vi "OEE_SCREEN_2_update_graph_accumulative_data.vi"(11 "SQL_raw_data_out":T1) -> ()   [LabVIEW 2019]
uses:
  FGV/SQL_raw_data/OEE_SQL_raw_data.ctl
  FGV/FGV_SCREEN_2_graph_accumulative/FGV_SCREEN_2_graph_accumulative.ctl
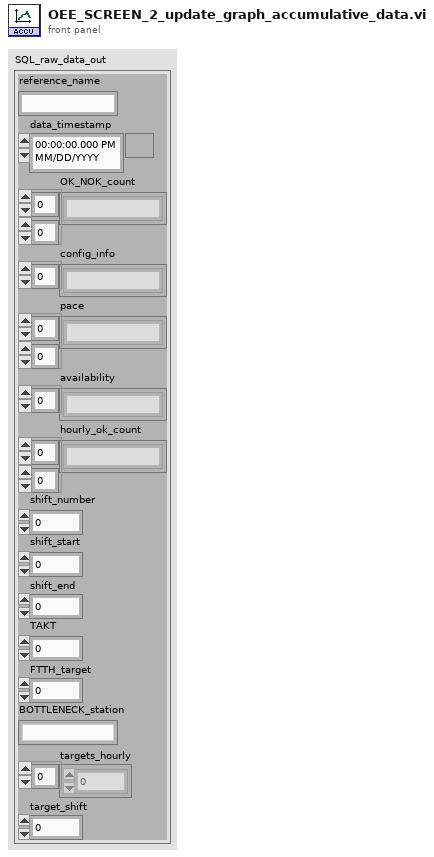
[diagram p1: front panel]
types:
  T1 = typedef "OEE_SQL_raw_data.ctl" = cluster{"reference_name":string, "data_timestamp":timestamp, "OK_NOK_count":string[][], "config_info":string[], "pace":string[][], "availability":string[], "hourly_ok_count":string[][], "shift_number":i8, "shift_start":i8, "shift_end":i8, "TAKT":u16, "FTTH_target":u16, "BOTTLENECK_station":string, "targets_hourly":u16[], "target_shift":u16}
  T2 = typedef "FGV_SCREEN_2_graph_accumulative.ctl" = enum16{"initialize", "set_hour_start", "set_hour_end", "set_target", "set_actual", "display"}
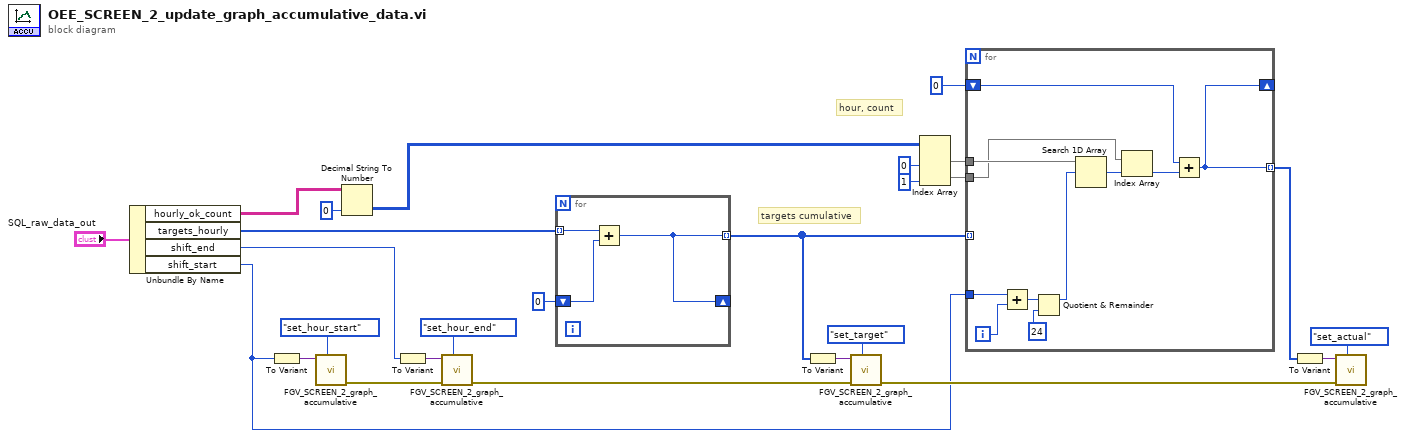
[diagram p0: block diagram]
diagram:
  # "hour, count"
  # "targets cumulative"
  n1 = Unbundle By Name("SQL_raw_data_out") -> ("hourly_ok_count"=w11:string[][], "targets_hourly"=w16:u16[], "shift_end"=w19:i8, "shift_start"=w4:i8)
  n2 = To Variant(anything=w4) -> (Variant=w21:variant)
  n3 = call "FGV_SCREEN_2_graph_accumulative.vi"("options"=FGV_SCREEN_2_graph_accumulative."set_hour_start", "input"=w21) -> ("error_out"=w20:errorcluster)  [unwired: 9 in]
  n4 = Decimal String To Number(string=w11, default (0L)=u16 0 ("default (0 I32)")) -> (number=w8:u16[][])  [unwired: 1 in, 1 out]
  n5 = To Variant(anything=w19) -> (Variant=w17:variant)
  n6 = call "FGV_SCREEN_2_graph_accumulative.vi"("options"=FGV_SCREEN_2_graph_accumulative."set_hour_end", "error_in"=w20, "input"=w17) -> ("error_out"=w13:errorcluster)  [unwired: 8 in]
  n7 = for {
    tunnel: w16 -> [w27] mode=indexing
    tunnel: [w29] -> w9 mode=indexing
    shift-right: [w29] -> _
    shift-left: u16 0 -> [w28]
    n8 = Add(x=w27, y=w28) -> (x+y=w29:u16)
  }
  n9 = To Variant(anything=w9) -> (Variant=w14:variant)
  n10 = call "FGV_SCREEN_2_graph_accumulative.vi"("options"=FGV_SCREEN_2_graph_accumulative."set_target", "error_in"=w13, "input"=w14) -> ("error_out"=w26:errorcluster)  [unwired: 8 in]
  n11 = Index Array(array=w8, index (col) #1=0 ("disabled index (col)"), index (col) #2=1 ("index (col)")) -> (element #1=w5:u16[], element #2=w3:u16[])  [unwired: 2 in]
  n12 = for {
    tunnel: w9 -> [_] mode=indexing
    tunnel: w5 -> [w38]
    tunnel: w4 -> [w39]
    tunnel: w3 -> [w36]
    tunnel: [w30] -> w2 mode=indexing
    shift-right: [w30] -> _
    shift-left: u16 0 -> [w31]
    i -> [w40]
    n13 = Add(x=w39, y=w40) -> (x+y=w35:i32)
    n14 = Quotient & Remainder(x=w35, y=24) -> (x-y*floor(x/y)=w33:i32)  [unwired: 1 out]
    n15 = Search 1D Array(1D array=w38, element=w33) -> (index of element=w37:i32)  [unwired: 1 in]
    n16 = Index Array(array=w36, index=w37) -> (element=w32:u16)
    n17 = Add(x=w31, y=w32) -> (x+y=w30:u16)
  }
  n18 = To Variant(anything=w2) -> (Variant=w12:variant)
  n19 = call "FGV_SCREEN_2_graph_accumulative.vi"("options"=FGV_SCREEN_2_graph_accumulative."set_actual", "error_in"=w26, "input"=w12) -> ()  [unwired: 8 in, 1 out]
